vi "Build Channel Tree.vi"(5 "Value Format":string, 7 "Tree":refnum<vi>, 11 "Groups":T1[](array[typedef])) -> ()   [LabVIEW 2020, in "VolatusDAQGenericGUI.lvlib"]
uses:
  VolatusDAQGenericGUI.lvlib
  Group Info.ctl
  lv-vecto/Vecto/Group/Group.lvclass
  AI Tree Entry.ctl
  Channel Entry.ctl
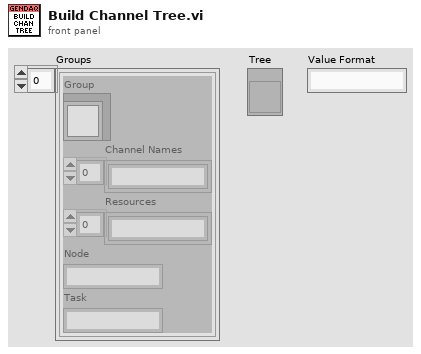
[diagram p1: front panel]
types:
  T1 = typedef "VolatusDAQGenericGUI.lvlib/Group Info.ctl" = cluster{"Group":refnum<class "Group.lvclass">, "Channel Names":string[], "Resources":string[], "Node":string, "Task":string}
  T2 = typedef "VolatusDAQGenericGUI.lvlib/AI Tree Entry.ctl" = cluster{"Hierarchy":string[], "Name":string, "Is Channel":bool, "Channel":T3}
  T3 = typedef "VolatusDAQGenericGUI.lvlib/Channel Entry.ctl" = cluster{"Resource":string, "Value":dbl, "Timestamp":dbl, "Raw":dbl}
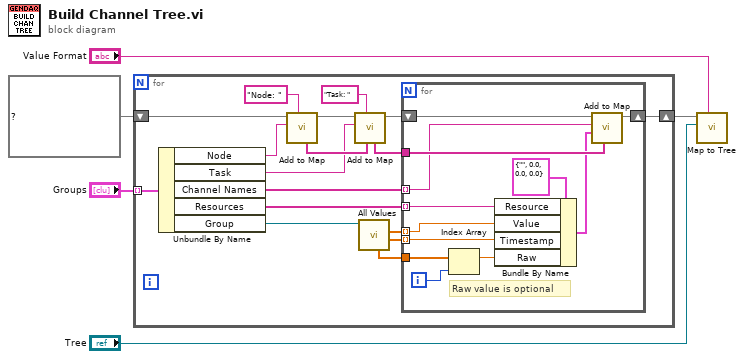
[diagram p0: block diagram]
diagram:
  n1 = for {
    shift-right: [w12] -> w4
    shift-left: map{string[], T2} {} ("Map in") -> [w22]
    tunnel: "Groups" -> [w11] mode=indexing
    n2 = Unbundle By Name(w11) -> ("Node"=w10:string, "Task"=w9:string, "Channel Names"=w6:string[], "Resources"=w8:string[], "Group"=w7:refnum<class "Group.lvclass">)
    n3 = call "Add to Map.vi"("Name Prefix (None)"="Node: ", "Name"=w10, "Map in"=w22) -> ("Map"=w20:map{string[], T2}, "Hierarchy"=w19:string[])  [unwired: 7 in]
    n4 = call "Add to Map.vi"("Parent (None)"=w19, "Name Prefix (None)"="Task: ", "Name"=w9, "Map in"=w20) -> ("Map"=w17:map{string[], T2}, "Hierarchy"=w16:string[])  [unwired: 6 in]
    n5 = call "All Values.vi"("Group in"=w7) -> ("Timestamp"=w14:dbl[], "Scaled"=w15:dbl[], "Raw"=w13:dbl[])  [unwired: 6 in, 2 out]
    n6 = for {
      shift-right: [w32] -> w12
      shift-left: w17 -> [w34]
      tunnel: w16 -> [w33]
      tunnel: w15 -> [w27] mode=indexing
      tunnel: w14 -> [w28] mode=indexing
      tunnel: w13 -> [w29]
      tunnel: w8 -> [w24] mode=indexing
      tunnel: w6 -> [w23] mode=indexing
      i -> [w25]
      # "Raw value is optional"
      n7 = Index Array(array=w29, index=w25) -> (element=w26:dbl)
      n8 = Bundle By Name(cluster=T3 {"Resource"="", "Value"=0.0, "Timestamp"=0.0, "Raw"=0.0} ("Channel (Not Channel)"), "Resource"=w24, "Value"=w27, "Timestamp"=w28, "Raw"=w26) -> (w30:T3)
      n9 = call "Add to Map.vi"("Parent (None)"=w33, "Channel (Not Channel)"=w30, "Name"=w23, "Map in"=w34) -> ("Map"=w32:map{string[], T2})  [unwired: 6 in, 1 out]
    }
  }
  n10 = call "Map to Tree.vi"("Value Format"="Value Format", "Tree"="Tree", "Map in"=w4) -> ()  [unwired: 9 in]
